vi "Register.vi"(8 "error in (no error)":errorcluster, 11 "Observer in":refnum<class "Observer.lvclass">) -> (0 "error out":errorcluster, 3 "Observer out":refnum<class "Observer.lvclass">)   [LabVIEW 2011, in "Observer.lvclass"]
uses:
  Observer.lvclass
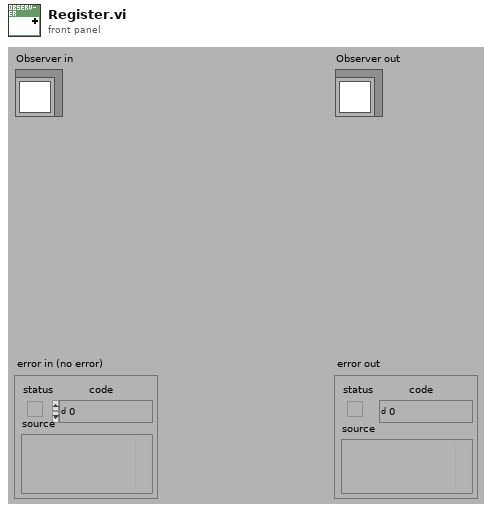
[diagram p1: front panel]
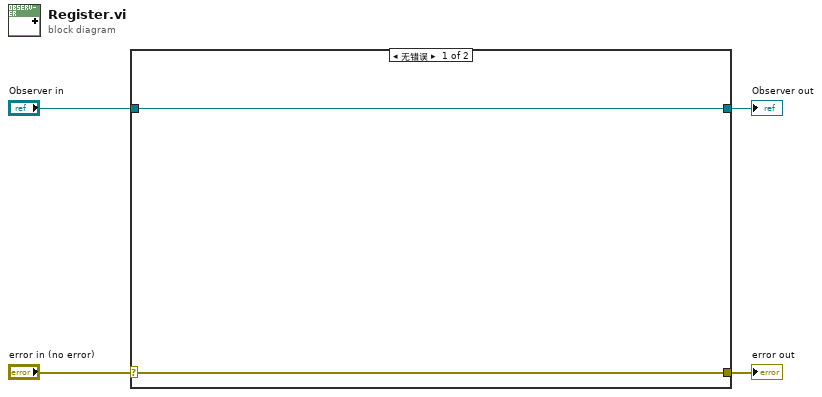
[diagram p0: block diagram]
diagram:
  n1 = case shown="无错误" "error in (no error)" {
    selector: "error in (no error)" -> [w5 w8]
    tunnel: [w5 w8] -> w1
    tunnel: [w6 w7] -> w3
    tunnel: "Observer in" -> [w6 w7]
    frame No Error {
    }
    frame Error {
    }
  }
  "Observer out" <- w3
  "error out" <- w1
